vi "Controller Select_Check Validity.vi"(4 "Software Version":u8, 6 "Controller?":bool, 7 "Unit ID (A)":string="A", 8 "error in":errorcluster, 9 "Controller Select_Old":u16(ring) items=["No controller"=0, "Volumetric Flow"=36, "Mass Flow"=37, "Absolute Pressure"=34, "Gauge Pressure"=38, "Differential Pressure"=39], 10 "Controller Select_New":u16(ring) items=["No controller"=0, "Volumetric Flow"=36, "Mass Flow"=37, "Absolute Pressure"=34, "Gauge Pressure"=38, "Differential Pressure"=39], 11 "VISA Session In":refnum<visa-resource-name>="Alicat") -> (0 "error out":errorcluster, 1 "Invalid selection":bool, 2 "Validated Controller Select":u16(ring) items=["No controller"=0, "Volumetric Flow"=36, "Mass Flow"=37, "Absolute Pressure"=34, "Gauge Pressure"=38, "Differential Pressure"=39], 3 "VISA Session Out":refnum<visa-resource-name>)   [LabVIEW 2014]
doc: "Checks the validity of a control variable selection. It will only return as valid if the variable is supported by the software and the unit is a controller. If using a controller, it will also report a variable selection of \"No Controller\" as invalid.\n\nIf unsupported or not a controller, this sub-VI will output the originally selected control variable as the validated selection."
uses:
  <vilib>/Instr/_visa.llb/VISA Flush IO Buffer Mask.ctl
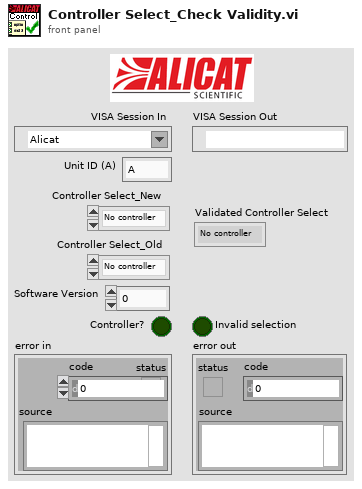
[diagram p1: front panel]
types:
  T1 = typedef "VISA Flush IO Buffer Mask.ctl" = u16
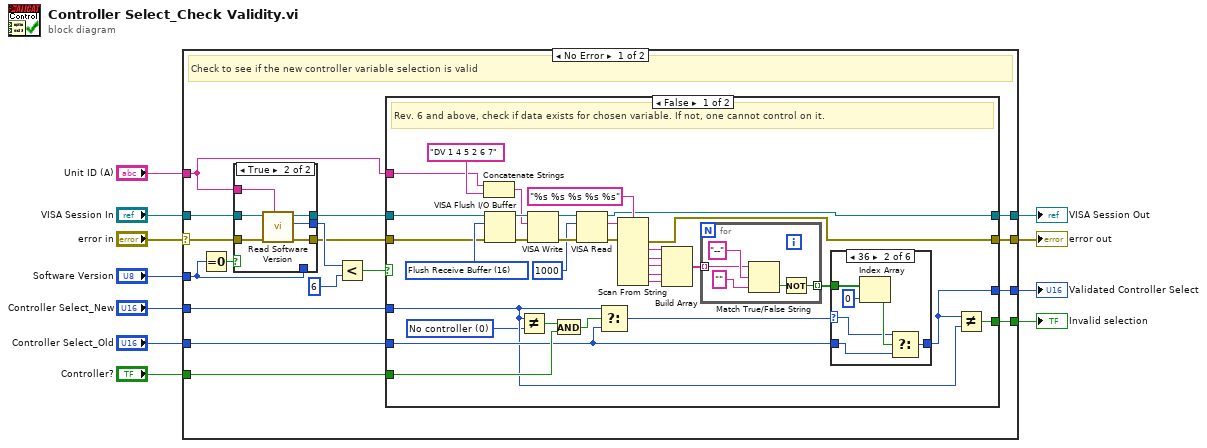
[diagram p0: block diagram]
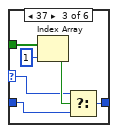
[diagram p4: hidden frame]
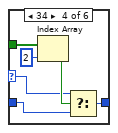
[diagram p5: hidden frame]
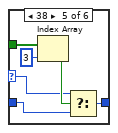
[diagram p6: hidden frame]
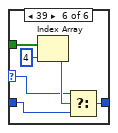
[diagram p7: hidden frame]
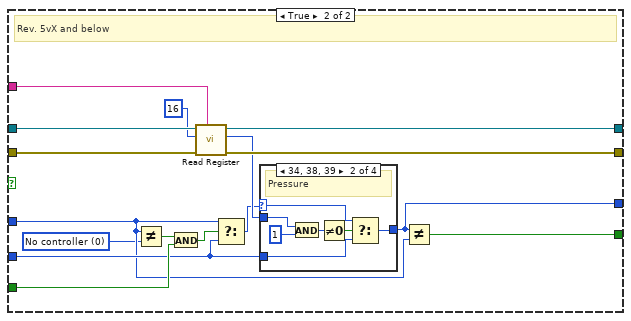
[diagram p8: hidden frame]
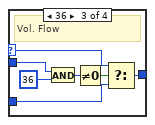
[diagram p10: hidden frame]
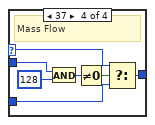
[diagram p11: hidden frame]
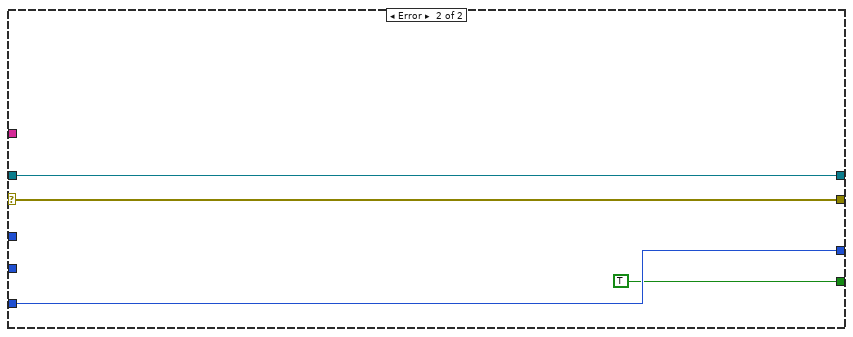
[diagram p12: hidden frame]
diagram:
  n1 = case shown="No Error" "error in" {
    selector: "error in" -> [w16 w142]
    tunnel: "VISA Session In" -> [w15 w144]
    tunnel: [w26 w142] -> w10
    tunnel: [w25 w144] -> w9
    tunnel: "Unit ID (A)" -> [w13 _]
    tunnel: "Controller Select_New" -> [w20 _]
    tunnel: "Controller?" -> [w24 _]
    tunnel: "Controller Select_Old" -> [w23 w145]
    tunnel: [w22 TRUE] -> w6
    tunnel: [w21 w145] -> w3
    tunnel: "Software Version" -> [w14 _]
    frame No Error {
      # "Check to see if the new controller variable selection is valid"
      n2 = Equal To 0?(x=w14) -> (x = 0?=w17:bool)
      n3 = case shown="True" w17 {
        tunnel: w16 -> [w28 w35]
        tunnel: w15 -> [w27 w34]
        tunnel: w13 -> [_ w33]
        tunnel: [w28 w32] -> _
        tunnel: [w27 w31] -> _
        tunnel: [w29 w30] -> w18
        tunnel: w14 -> [w29 _]
        frame False {
        }
        frame True {
          n4 = call "Read Software Version.vi"("Unit ID (A)"=w33, "error in"=w35, "VISA Session In"=w34) -> ("error out"=w32:errorcluster, "Software Version"=w30:u8, "VISA Session Out"=w31:refnum<visa-resource-name>)  [unwired: 6 in]
        }
      }
      n5 = Less?(x=w18, y=u8 6) -> (x < y?=w12:bool)
      n6 = case shown="False" w12 {
        tunnel: w15 -> [w38 w117]
        tunnel: [w46 w116] -> w26
        tunnel: [w48 w115] -> w25
        tunnel: w13 -> [w45 w114]
        tunnel: w24 -> [w65 w112]
        tunnel: w23 -> [w42 w109]
        tunnel: [w41 w108] -> w22
        tunnel: [w40 w107] -> w21
        tunnel: w16 -> [w37 w106]
        tunnel: w20 -> [w39 w105]
        frame False {
          w36 = u16 0 items=["No controller"=0, "Volumetric Flow"=36, "Mass Flow"=37, "Absolute Pressure"=34, "Gauge Pressure"=38, "Differential Pressure"=39] ("Controller Select")
          w53 = T1 16 items=["Flush Receive Buffer"=16, "Write Transmit Buffer to Device"=32, "Flush Receive Buffer (No I/O)"=64, "Flush Transmit Buffer"=128] ("Mask")
          # "Rev. 6 and above, check if data exists for chosen variable. If not, one cannot control on it."
          n7 = Concatenate Strings(w45, "DV 1 4 5 2 6 7" ("string")) -> (w49:string)
          n8 = VISA Flush I/O Buffer(VISA resource name=w38, mask (16)=w53, error in (no error)=w37) -> (VISA resource name out=w52:refnum<visa-resource-name>, error out=w51:errorcluster)
          n9 = Not Equal?(x=w39, y=w36) -> (x != y?=w67:bool)
          n10 = VISA Write(VISA resource name=w52, write buffer=w49, error in (no error)=w51) -> (VISA resource name out=w55:refnum<visa-resource-name>, error out=w56:errorcluster)  [unwired: 1 out]
          n11 = And(x=w67, y=w65) -> (x .and. y?=w66:bool)
          n12 = VISA Read(VISA resource name=w55, byte count=u32 1000, error in (no error)=w56) -> (VISA resource name out=w48:refnum<visa-resource-name>, read buffer=w64:string, error out=w47:errorcluster)  [unwired: 1 out]
          n13 = Select(t=w39, s=w66, f=w42) -> (s? t:f=w43:u16)
          n14 = Scan From String(format string="%s %s %s %s %s", input string=w64, error in=w47) -> (error out=w46:errorcluster, output 1=w58:string, output 2=w59:string, output 3=w60:string, output 4=w61:string, output 5=w62:string)  [unwired: 6 in, 2 out]
          n15 = Build Array(w58, w59, w60, w61, w62) -> (w63:string[])
          n16 = for {
            tunnel: w63 -> [w101] mode=indexing
            tunnel: [w99] -> w44 mode=indexing
            n17 = Match True/False String(2:"" ("false string"), 3:"--", 4:w101) -> (0:w100:bool)  [unwired: 1 out]
            n18 = Not(x=w100) -> (.not. x?=w99:bool)
          }
          n19 = case shown="36" w43 {
            selector: w43 -> [w68 w71 w77 w83 w89 w95]
            tunnel: w44 -> [_ w74 w80 w86 w92 w98]
            tunnel: w42 -> [_ w70 w76 w82 w88 w94]
            tunnel: [w68 w69 w75 w81 w87 w93] -> w40
            frame 0, Default {
            }
            frame 36 {
              n20 = Index Array(array=w74, index=0) -> (element=w73:bool)
              n21 = Select(t=w71, s=w73, f=w70) -> (s? t:f=w69:u16)
            }
            frame 37 {
              n22 = Index Array(array=w80, index=1) -> (element=w79:bool)
              n23 = Select(t=w77, s=w79, f=w76) -> (s? t:f=w75:u16)
            }
            frame 34 {
              n24 = Index Array(array=w86, index=2) -> (element=w85:bool)
              n25 = Select(t=w83, s=w85, f=w82) -> (s? t:f=w81:u16)
            }
            frame 38 {
              n26 = Index Array(array=w92, index=3) -> (element=w91:bool)
              n27 = Select(t=w89, s=w91, f=w88) -> (s? t:f=w87:u16)
            }
            frame 39 {
              n28 = Index Array(array=w98, index=4) -> (element=w97:bool)
              n29 = Select(t=w95, s=w97, f=w94) -> (s? t:f=w93:u16)
            }
          }
          n30 = Not Equal?(x=w40, y=w39) -> (x != y?=w41:bool)
        }
        frame True {
          w104 = u16 0 items=["No controller"=0, "Volumetric Flow"=36, "Mass Flow"=37, "Absolute Pressure"=34, "Gauge Pressure"=38, "Differential Pressure"=39] ("Controller Select")
          # "Rev. 5vX and below"
          n31 = Not Equal?(x=w105, y=w104) -> (x != y?=w119:bool)
          n32 = And(x=w119, y=w112) -> (x .and. y?=w118:bool)
          n33 = call "Read Register.vi"("Unit ID (A)"=w114, "error in"=w106, "Register address"=u16 16, "VISA Session In"=w117) -> ("error out"=w116:errorcluster, "Register Value (I32)"=w111:i32, "VISA Session Out"=w115:refnum<visa-resource-name>)  [unwired: 5 in]
          n34 = Select(t=w105, s=w118, f=w109) -> (s? t:f=w110:u16)
          n35 = case shown="34, 38, 39" w110 {
            selector: w110 -> [w120 w125 w131 w137]
            tunnel: w111 -> [_ w126 w128 w135]
            tunnel: w109 -> [_ w124 w130 w138]
            tunnel: [w120 w122 w129 w136] -> w107
            frame 0, Default {
              # "No Controller"
            }
            frame 34, 38, 39 {
              # "Pressure"
              n36 = And(x=w126, y=1) -> (x .and. y?=w123:i32)
              n37 = Not Equal To 0?(x=w123) -> (x != 0?=w121:bool)
              n38 = Select(t=w125, s=w121, f=w124) -> (s? t:f=w122:u16)
            }
            frame 36 {
              # "Vol. Flow"
              n39 = And(x=w128, y=36) -> (x .and. y?=w133:i32)
              n40 = Not Equal To 0?(x=w133) -> (x != 0?=w132:bool)
              n41 = Select(t=w131, s=w132, f=w130) -> (s? t:f=w129:u16)
            }
            frame 37 {
              # "Mass Flow"
              n42 = And(x=w135, y=128) -> (x .and. y?=w140:i32)
              n43 = Not Equal To 0?(x=w140) -> (x != 0?=w139:bool)
              n44 = Select(t=w137, s=w139, f=w138) -> (s? t:f=w136:u16)
            }
          }
          n45 = Not Equal?(x=w107, y=w105) -> (x != y?=w108:bool)
        }
      }
    }
    frame Error {
    }
  }
  "error out" <- w10
  "VISA Session Out" <- w9
  "Invalid selection" <- w6
  "Validated Controller Select" <- w3
